vi "pwm_test.vi"() -> ()   [LabVIEW 2019]
uses:
  <vilib>/DAQmx/create/channels.llb/DAQmx Create Channel (CO-Pulse Generation-Frequency).vi
  <vilib>/DAQmx/configure/timing.llb/DAQmx Timing (Implicit).vi
  <vilib>/DAQmx/write.llb/DAQmx Write (Counter Frequency 1Chan 1Samp).vi
  <vilib>/Utility/error.llb/DialogType.ctl
panel:
  in  "Stop":bool
  in  "Counter":tag="Dev1/ctr0"
  in  "Frequency":dbl=1.0 format="%.6f"
  in  "Duty Cycle":dbl=0.5 format="%.6f"
  in  "Iniital Delay":dbl format="%.6f"
  in  "Idle State":i32(ring)=10214 items=["High"=10192, "Low"=10214]
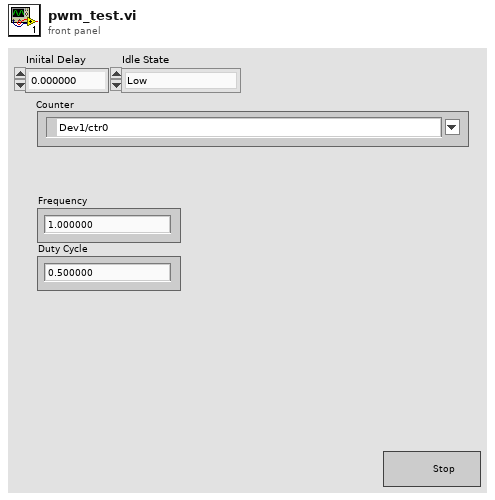
[diagram p1: front panel]
types:
  T1 = typedef "DialogType.ctl" = u16
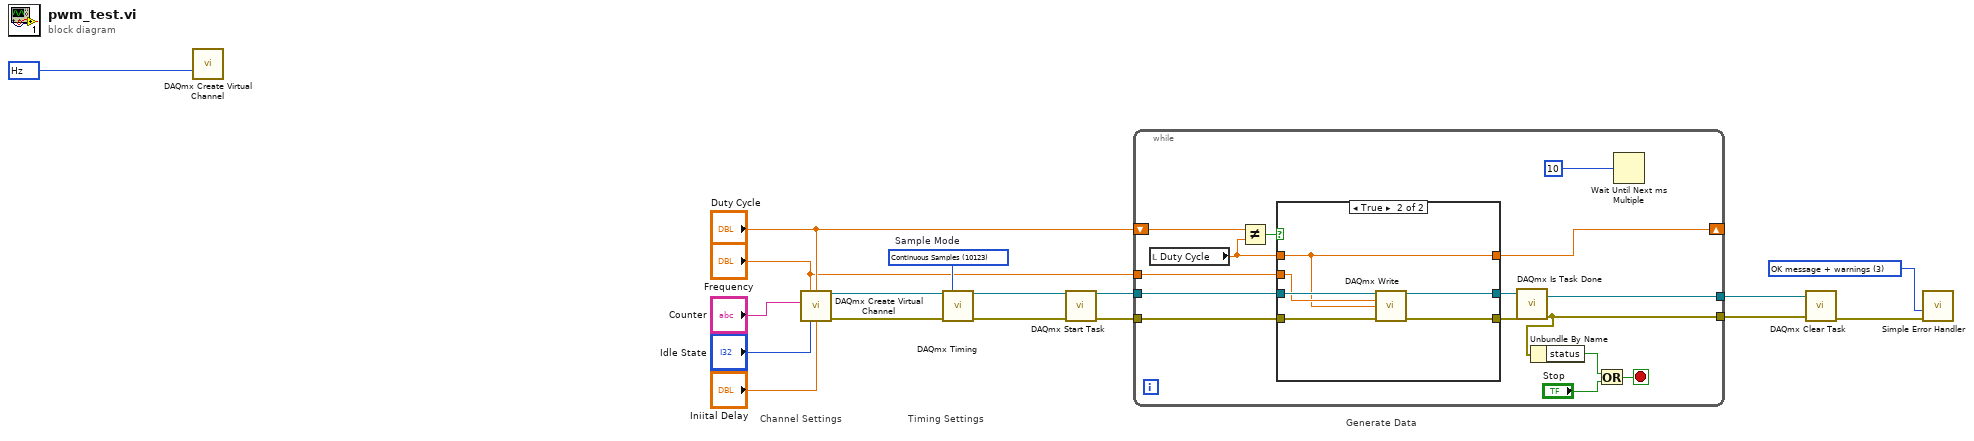
[diagram p0: block diagram]
diagram:
  w11 = T1 3 items=["no dialog", "OK message", "continue or stop message", "OK message + warnings", "continue/stop + warnings"] ("type of dialog (OK msg:1)")
  w16 = 10123 items=["Finite Samples"=10178, "Continuous Samples"=10123, "Hardware Timed Single Point"=12522]  # Sample Mode
  w17 = 10373 items=["Hz"=10373] ("units")
  # "Generate Data"
  # "Timing Settings"
  # "Channel Settings"
  n1 = call-poly <vilib>:"DAQmx Create Virtual Channel.vi"("units"=w17) -> ()  [unwired: 13 in, 2 out]
  n2 = call-poly <vilib>:"DAQmx Create Virtual Channel.vi"("frequency"="Frequency", "duty cycle"="Duty Cycle", "counter"="Counter", "idle state"="Idle State", "initial delay"="Iniital Delay") -> ("task out"=w8:refnum<k21>, "error out"=w7:errorcluster)  [unwired: 9 in]
  n3 = call-poly <vilib>:"DAQmx Timing.vi"("task/channels in"=w8, "sample mode"=w16, "error in"=w7) -> ("task out"=w6:refnum<k21>, "error out"=w5:errorcluster)  [unwired: 11 in]
  n4 = call <vilib>:"DAQmx Start Task.vi"("task/channels in"=w6, "error in"=w5) -> ("task out"=w15:refnum<k21>, "error out"=w14:errorcluster)  [unwired: 12 in]
  n5 = while {
    tunnel: w15 -> [w24]
    tunnel: w14 -> [w23]
    tunnel: [w26] -> w4
    tunnel: [w25] -> w3
    tunnel: "Frequency" -> [w19]
    shift-right: [w18] -> _
    shift-left: "Duty Cycle" -> [w22]
    stop <- w32 stop-if-true
    n6 = local read "Duty Cycle"() -> (w21:dbl)
    n7 = Not Equal?(x=w22, y=w21) -> (x != y?=w20:bool)
    n8 = case shown="True" w20 {
      tunnel: w23 -> [w33 w41]
      tunnel: w24 -> [w34 w40]
      tunnel: [w34 w39] -> w28
      tunnel: [w33 w38] -> w27
      tunnel: w21 -> [w35 w36]
      tunnel: w19 -> [_ w37]
      tunnel: [w35 w36] -> w18
      frame False {
      }
      frame True {
        n9 = call-poly <vilib>:"DAQmx Write.vi"("task/channels in"=w40, "frequency"=w37, "duty cycle"=w36, "error in"=w41) -> ("task out"=w39:refnum<k21>, "error out"=w38:errorcluster)  [unwired: 9 in, 1 out]
      }
    }
    n10 = call <vilib>:"DAQmx Is Task Done.vi"("task/channels in"=w28, "error in"=w27) -> ("task out"=w25:refnum<k21>, "error out"=w26:errorcluster)  [unwired: 11 in, 1 out]
    n11 = Unbundle By Name(w26) -> ("status"=w31:bool)
    n12 = Or(x=w31, y="Stop") -> (x .or. y?=w32:bool)
    n13 = Wait Until Next ms Multiple(millisecond multiple=u32 10) -> ()  [unwired: 1 out]
  }
  n14 = call <vilib>:"DAQmx Clear Task.vi"("task in"=w3, "error in"=w4) -> ("error out"=w13:errorcluster)  [unwired: 13 in]
  n15 = call <vilib>:"Simple Error Handler.vi"("type of dialog (OK msg:1)"=w11, "error in (no error)"=w13) -> ()  [unwired: 3 in, 5 out]
